vi "HandleResponse.vi"(8 "error in (no error)":errorcluster, 10 "response":T1, 11 "PolledDriver in":refnum<class "PolledDriver.lvclass">) -> (0 "error out":errorcluster, 2 "Response out":T1[](array[typedef]), 3 "PolledDriver out":refnum<class "PolledDriver.lvclass">)   [LabVIEW 2013, in "PolledDriver.lvclass"]
doc: "Callback for any responses retreived from the remote destination. Overload this method to do any special handling in your driver"
uses:
  PolledDriver.lvclass
  response.ctl
  driver_status.ctl
  BaseDriver/BaseDriver.lvclass
  PolledDriver.lvclass/PolledDriver.ctl
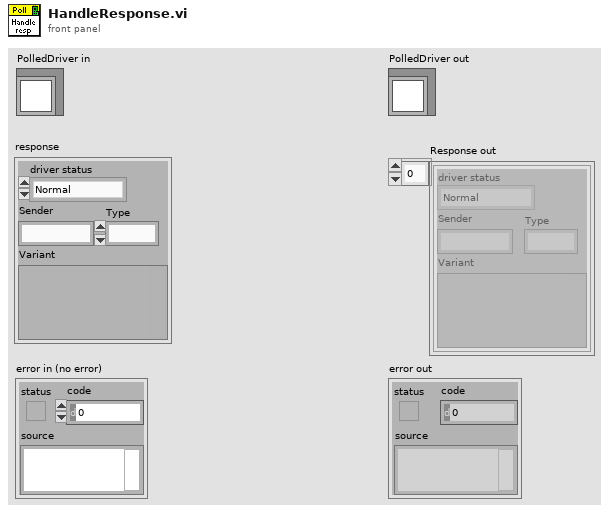
[diagram p1: front panel]
types:
  T1 = typedef "response.ctl" = cluster{"driver status":T2, "Sender":string, "Type":i32, "Variant":variant}
  T2 = typedef "driver_status.ctl" = enum16{"Normal", "Startup", "Connection lost", "Reconnected", "Timeout", "Idle", "Busy"}
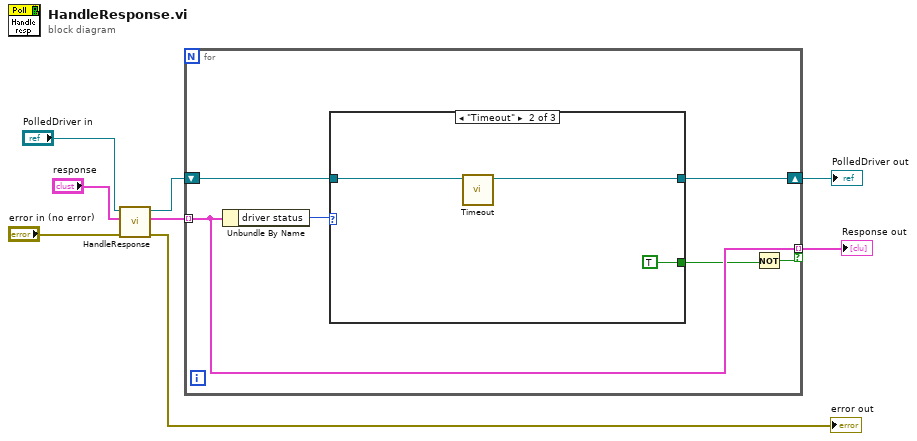
[diagram p0: block diagram]
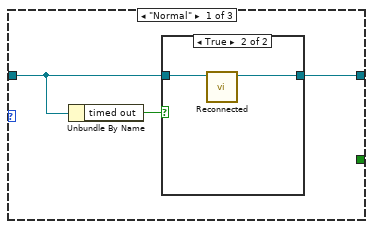
[diagram p2: hidden frame]
diagram:
  n1 = call-parent "HandleResponse.vi"("error in (no error)"="error in (no error)", "response"="response", "BaseDriver in"="PolledDriver in") -> ("error out"=→"error out":errorcluster, "Response out"=w8:T1[], "BaseDriver out"=w7:refnum<class "PolledDriver.lvclass">)  [unwired: 6 in]
  n2 = for {
    tunnel: w8 -> [w11] mode=indexing
    shift-right: [w12] -> w2
    shift-left: w7 -> [w13]
    tunnel: [w11] -> w3 mode=indexing if=w9
    n3 = Unbundle By Name(w11) -> ("driver status"=w14:T2)
    n4 = case shown="\"Timeout\"" w14 {
      tunnel: w13 -> [w16 w23 w24]
      tunnel: [w15 w22 w24] -> w12
      tunnel: [_ TRUE _] -> w10
      frame "Normal" {
        n5 = Unbundle By Name(w16) -> ("timed out"=w17:bool)
        n6 = case shown="True" w17 {
          tunnel: w16 -> [w18 w20]
          tunnel: [w18 w19] -> w15
          frame False {
          }
          frame True {
            n7 = call "Reconnected.vi"("PolledDriver in"=w20) -> ("PolledDriver out"=w19:refnum<class "PolledDriver.lvclass">)  [unwired: 9 in, 1 out]
          }
        }
      }
      frame "Timeout" {
        n8 = call-dynamic "Timeout.vi"("PolledDriver in"=w23) -> ("PolledDriver out"=w22:refnum<class "PolledDriver.lvclass">)  [unwired: 8 in, 2 out]
      }
      frame "Idle", Default {
      }
    }
    n9 = Not(x=w10) -> (.not. x?=w9:bool)
  }
  "Response out" <- w3
  "PolledDriver out" <- w2
